vi "PCE_ANSWER-error-handler(bol-array).vi"(1 "Serial?":bool, 2 "Boolean array":bool[](array[boolean])) -> (0 "PCE answer":string)   [LabVIEW 2010]
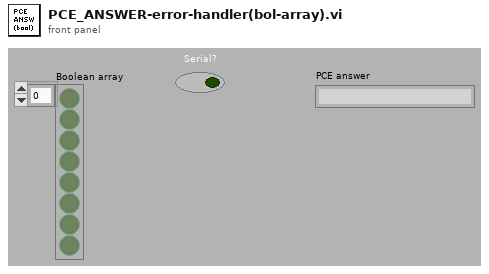
[diagram p1: front panel]
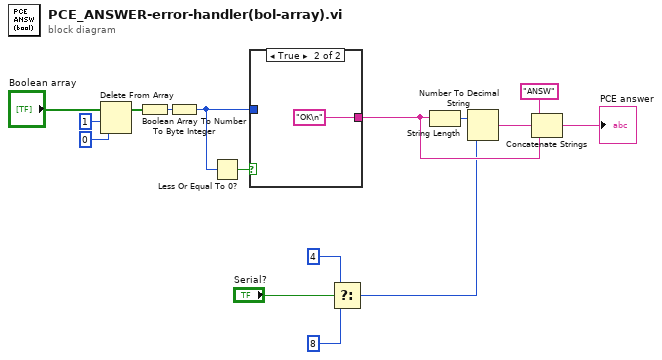
[diagram p0: block diagram]
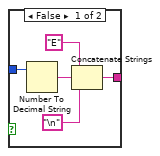
[diagram p2: hidden frame]
diagram:
  n1 = Delete From Array(array="Boolean array", length=1, index=0) -> (array with subset deleted=w5:bool[])  [unwired: 1 out]
  n2 = Boolean Array To Number(Boolean array=w5) -> (number=w14:u32)
  n3 = To Byte Integer(number=w14) -> (8bit integer=w6:i8)
  n4 = Less Or Equal To 0?(x=w6) -> (x <= 0?=w7:bool)
  n5 = case shown="True" w7 {
    tunnel: w6 -> [w19 _]
    tunnel: [w18 "OK\n"] -> w10
    frame False {
      n6 = Number To Decimal String(number=w19) -> (decimal integer string=w21:string)  [unwired: 1 in]
      n7 = Concatenate Strings("E" ("string"), w21, "\n" ("string")) -> (w18:string)
    }
    frame True {
    }
  }
  n8 = Select(t=i16 4 ("width (-)"), s="Serial?", f=i16 8 ("width (-)")) -> (s? t:f=w1:i16)
  n9 = String Length(string=w10) -> (length=w11:i32)
  n10 = Number To Decimal String(number=w11, width (-)=w1) -> (decimal integer string=w9:string)
  n11 = Concatenate Strings("ANSW" ("string"), w9, w10) -> (→"PCE answer":string)
